vi "Icon Create Header.vi"() -> ()   [LabVIEW 2018]
uses:
  <vilib>/picture/picture.llb/imagedata.ctl
panel:
  out "Color256":T1
  in  "Text":string
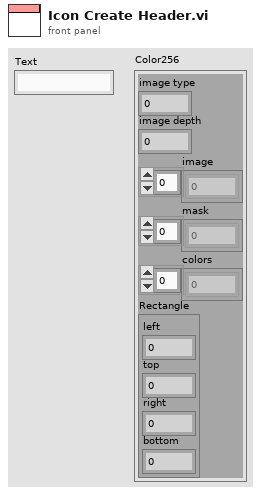
[diagram p1: front panel]
types:
  T1 = typedef "imagedata.ctl" = cluster{"image type":i32, "image depth":i32, "image":u8[], "mask":u8[], "colors":u32[], "Rectangle":cluster{"left":i16, "top":i16, "right":i16, "bottom":i16}}
  T2 = cluster{"left":i16, "top":i16, "right":i16, "bottom":i16}
  T3 = cluster{"Font Name:":string, "Size":i16, "Strikeout?":bool, "Italic?":bool, "Underline?":bool, "Outline?":bool, "Shadow?":bool, "Bold?":bool}
  T4 = enum16{"User-specified Font", "Application Font", "System Font", "Dialog Font"}
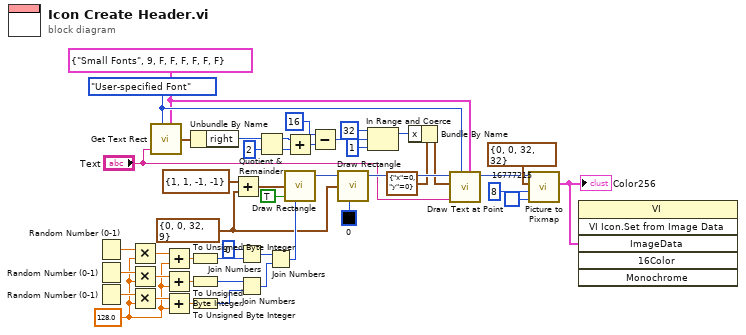
[diagram p0: block diagram]
diagram:
  w11 = 128.0 ("y")
  w24 = T2 {"left"=0, "top"=0, "right"=32, "bottom"=9} ("rect")
  w21 = T3 {"Font Name:"="Small Fonts", "Size"=9, "Strikeout?"=FALSE, "Italic?"=FALSE, "Underline?"=FALSE, "Outline?"=FALSE, "Shadow?"=FALSE, "Bold?"=FALSE} ("[user-specified font]")
  w22 = T4."User-specified Font" ("desired font(Application)")
  n1 = Random Number (0-1)() -> (number: 0 to 1=w40:dbl)
  n2 = Random Number (0-1)() -> (number: 0 to 1=w39:dbl)
  n3 = Random Number (0-1)() -> (number: 0 to 1=w36:dbl)
  n4 = Multiply(x=w40, y=w11) -> (x*y=w41:dbl)
  n5 = Multiply(x=w39, y=w11) -> (x*y=w38:dbl)
  n6 = Multiply(x=w36, y=w11) -> (x*y=w37:dbl)
  n7 = call <vilib>:"Get Text Rect.vi"("desired font(Application)"=w22, "text"="Text", "[user-specified font]"=w21) -> ("rect"=w20:T2)  [unwired: 6 in]
  n8 = Add(x=w41, y=w11) -> (x+y=w12:dbl)
  n9 = Add(x=w38, y=w11) -> (x+y=w13:dbl)
  n10 = Add(x=w37, y=w11) -> (x+y=w14:dbl)
  n11 = To Unsigned Byte Integer(number=w12) -> (unsigned 8bit integer=w35:u8)
  n12 = To Unsigned Byte Integer(number=w13) -> (unsigned 8bit integer=w33:u8)
  n13 = To Unsigned Byte Integer(number=w14) -> (unsigned 8bit integer=w32:u8)
  n14 = Unbundle By Name(w20) -> ("right"=w5:i16)
  n15 = Add(x=T2 {"left"=1, "top"=1, "right"=-1, "bottom"=-1} ("rect"), y=w24) -> (x+y=w25:T2)
  n16 = Join Numbers(hi=u8 0, lo=w35) -> ((hi.lo)=w30:u16)
  n17 = Join Numbers(hi=w33, lo=w32) -> ((hi.lo)=w31:u16)
  n18 = Quotient & Remainder(x=w5, y=i16 2) -> (x-y*floor(x/y)=w2:i16, floor(x/y)=w8:i16)
  n19 = Join Numbers(hi=w30, lo=w31) -> ((hi.lo)=w29:u32)
  n20 = Add(x=w2, y=w8) -> (x+y=w3:i16)
  n21 = call <vilib>:"Draw Rectangle.vi"("rect"=w25, "fill?(F)"=TRUE, "color(black)"=w29) -> ("new picture"=w43:picture)  [unwired: 6 in]
  n22 = Subtract(x=i16 16 ("y"), y=w3) -> (x-y=w1:i16)
  n23 = call <vilib>:"Draw Rectangle.vi"("picture"=w43, "rect"=w24, "color(black)"=u32 0) -> ("new picture"=w23:picture)  [unwired: 6 in]
  n24 = In Range and Coerce(upper limit=i16 32, x=w1, lower limit=i16 1) -> (coerced(x)=w7:i16)  [unwired: 1 out]
  n25 = Bundle By Name(cluster=cluster{"x":i16, "y":i16} {"x"=0, "y"=0} ("origin"), "x"=w7) -> (w17:cluster{"x":i16, "y":i16})
  n26 = call <vilib>:"Draw Text at Point.vi"("[user-specified font]"=w21, "desired font(Application)"=w22, "text"="Text", "origin"=w17, "picture"=w23) -> ("new picture"=w16:picture)  [unwired: 5 in, 1 out]
  n27 = call <vilib>:"Picture to Pixmap.vi"("Background Color"=u32 16777215, "depth"=8, "rect"=T2 {"left"=0, "top"=0, "right"=32, "bottom"=32}, "picture"=w16) -> ("image data"=w6:T1)  [unwired: 6 in, 1 out]
  "Color256" <- w6
  n28 = invoke class="VI" method="VI Icon.Set from Image Data"("ImageData"=w6) -> ()  [unwired: 5 in, 6 out]
